vi "菜单-打开.vi"(8 "error in (no error)":errorcluster caption="错误输入（无错误）", 11 "程序响应 输入":refnum<class "程序响应.lvclass">) -> (0 "error out":errorcluster caption="错误输出", 3 "程序响应 输出":refnum<class "程序响应.lvclass">)   [LabVIEW 2018, in "程序响应.lvlib" / "程序响应.lvclass"]
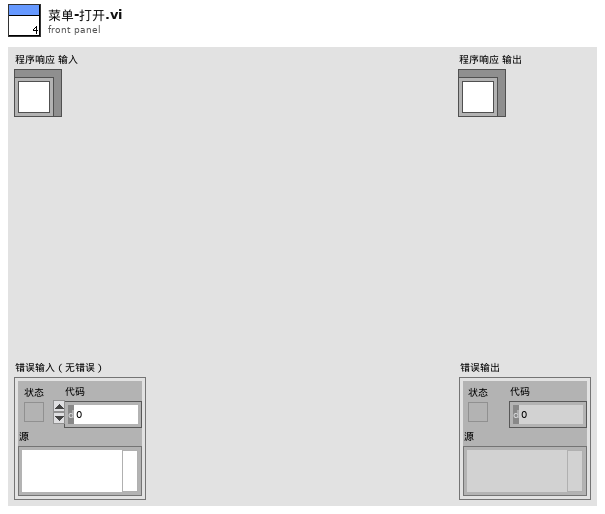
[diagram p1: front panel]
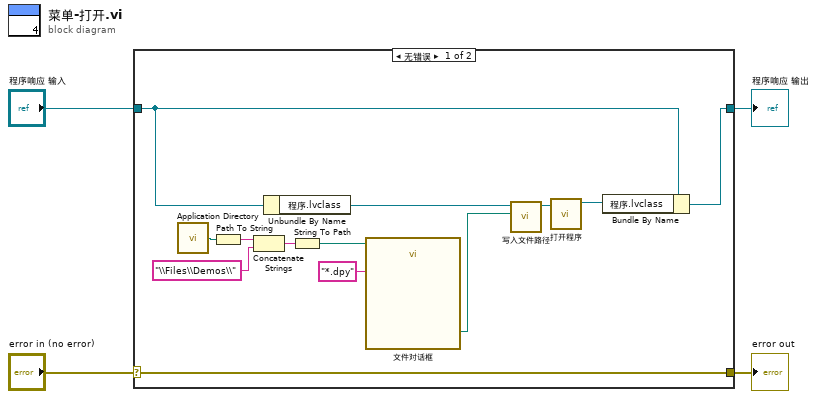
[diagram p0: block diagram]
diagram:
  n1 = case shown="无错误" "error in (no error)" {
    selector: "error in (no error)" -> [w17 w19]
    tunnel: [w17 w19] -> w3
    tunnel: [w14 w18] -> w1
    tunnel: "程序响应 输入" -> [w15 w18]
    frame No Error {
      n2 = call <vilib>:"Application Directory.vi"() -> ("Application Directory"=w6:path)
      n3 = Path To String(path=w6) -> (string=w9:string)
      n4 = Concatenate Strings(w9, "\\Files\\Demos\\" ("名称或相对路径")) -> (w8:string)
      n5 = Unbundle By Name(w15) -> ("程序.lvclass"=w13:refnum<class "程序.lvclass">)
      n6 = String To Path(string=w8) -> (path=w5:path)
      n7 = call "文件对话框"("start path"=w5, "pattern (all files)"="*.dpy") -> ("selected path"=w11:path)  [unwired: 10 in, 3 out]
      n8 = call-dynamic "写入文件路径.vi"("文件路径"=w11, "程序输入"=w13) -> ("程序输出"=w12:refnum<class "程序.lvclass">)  [unwired: 8 in, 1 out]
      n9 = call-dynamic "打开程序.vi"("程序 输入"=w12) -> ("程序 输出"=w16:refnum<class "程序.lvclass">)  [unwired: 9 in, 1 out]
      n10 = Bundle By Name(cluster=w15, "程序.lvclass"=w16) -> (w14:refnum<class "程序响应.lvclass">)
    }
    frame Error {
    }
  }
  "error out" <- w3
  "程序响应 输出" <- w1
